vi "Zip Files.vi"(8 "error in (no error)":errorcluster, 10 "Source File/Directory":path, 11 "Target Zip File":path) -> (0 "error out":errorcluster, 3 "Path to .zip":path)   [LabVIEW 2011]
doc: "This VI will zip-up a Source File or Directory into the Target Zip File.\n\nInstructions:\n1) Run the VI\n2) Select a zip file that you want to create or overwrite (Target Zip File).\n3) Select either a file or directory that you want to compress (Source File/Directory)."
panel:
  # "This VI will zip-up a Source File or Directory into the Target Zip File.\n\nInstructions:\n1) Run the VI\n2) Select a zip file that you want to create or overwrite (Target Zip File).\n3) Select either a file or directory that you want to compress (Source File/Directory)."
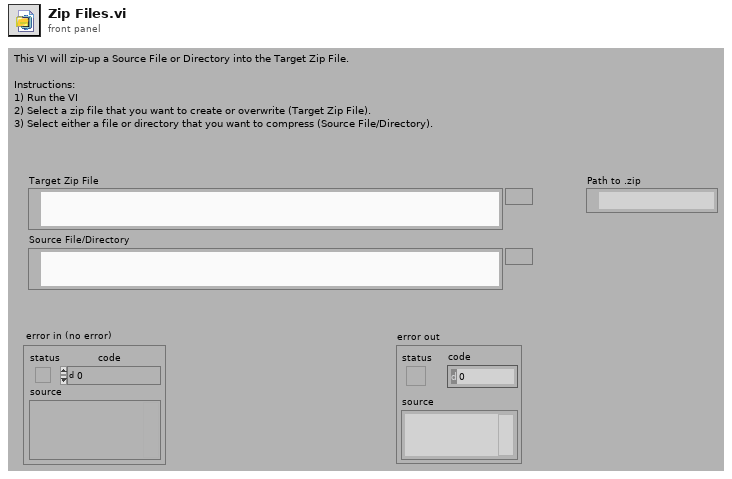
[diagram p1: front panel]
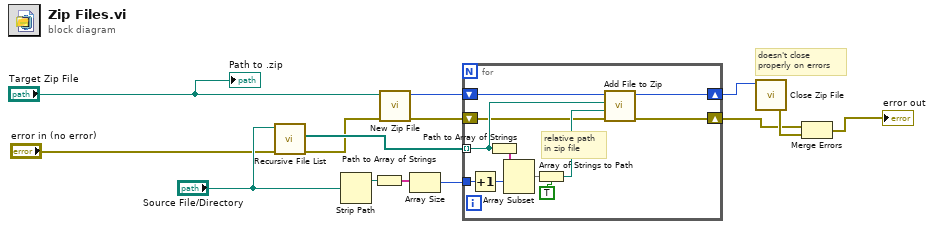
[diagram p0: block diagram]
diagram:
  # "doesn't close\nproperly on errors"
  n1 = call <vilib>:"Recursive File List.vi"("error in (no error)"="error in (no error)", "Folder Path"="Source File/Directory") -> ("error out"=w7:errorcluster, "All Files in Dir"=w9:path[])  [unwired: 1 in, 7 out]
  n2 = Strip Path(path="Source File/Directory") -> (stripped path=w13:path)  [unwired: 1 out]
  n3 = Path to Array of Strings(0:w13) -> (2:w12:string[])  [unwired: 1 out]
  n4 = call <vilib>:"New Zip File.vi"("error in (no error)"=w7, "target"="Target Zip File") -> ("error out"=w4:errorcluster, "zip file out"=w6:i64)  [unwired: 1 in, 3 out]
  n5 = Array Size(array=w12) -> (size(s)=w11:i32)
  n6 = for {
    tunnel: w9 -> [w25] mode=indexing
    tunnel: w11 -> [w23]
    shift-right: [w15] -> w3
    shift-left: w6 -> [w16]
    shift-right: [w18] -> w2
    shift-left: w4 -> [w17]
    # "relative path\nin zip file"
    n7 = Increment(x=w23) -> (x+1=w19:i32)
    n8 = Path to Array of Strings(0:w25) -> (2:w24:string[])  [unwired: 1 out]
    n9 = Array Subset(array=w24, index=w19) -> (w22:string[])  [unwired: 1 in]
    n10 = Array of Strings to Path(0:w22, 1:TRUE ("relative")) -> (2:w21:path)
    n11 = call <vilib>:"Add File to Zip.vi"("error in (no error)"=w17, "destination path in zip"=w21, "source file path"=w25, "zip file in"=w16) -> ("error out"=w18:errorcluster, "zip file out"=w15:i64)  [unwired: 6 out]
  }
  n12 = call <vilib>:"Close Zip File.vi"("zip file in"=w3) -> ("error out"=w5:errorcluster)  [unwired: 2 in, 4 out]
  n13 = Merge Errors(w2, w5) -> (→"error out":errorcluster)
  "Path to .zip" <- "Target Zip File"
